vi "FilesIOex1.vi"() -> ()   [LabVIEW 2015]
panel:
  in  "access (0:read/write)":enum16{"read/write", "read-only", "write-only"}(ring)
  in  "operation (0:open)":T1(ring)
  in  "stop":bool
  in  "file path (use dialog)":path
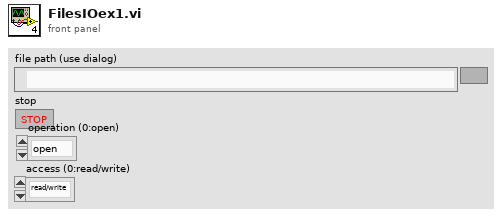
[diagram p1: front panel]
types:
  T1 = enum16{"open", "replace", "create", "open or create", "replace or create", "replace or create with confirmation"}
  T2 = enum16{"Native", "Native Command Line", "UNIX", "Macintosh", "DOS"}
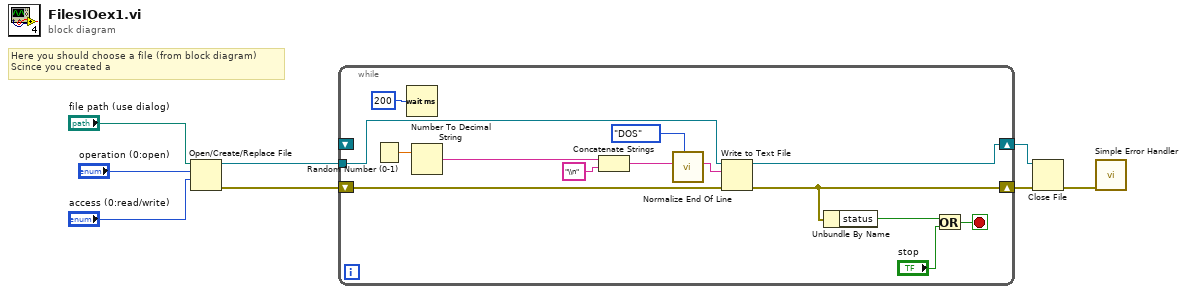
[diagram p0: block diagram]
diagram:
  # "Here you should choose a file (from block diagram)\nScince you created a"
  n1 = Open/Create/Replace File(file path (use dialog)="file path (use dialog)", operation (0:open)="operation (0:open)", access (0:read/write)="access (0:read/write)") -> (refnum out=w7:refnum<file>, error out=w6:errorcluster)  [unwired: 3 in, 1 out]
  n2 = while {
    tunnel: w7 -> [w18]
    shift-right: [w17] -> w4
    shift-left: _ -> [_]
    shift-right: [w15] -> w5
    shift-left: w6 -> [w16]
    stop <- w22 stop-if-true
    n3 = Random Number (0-1)() -> (number: 0 to 1=w19:dbl)
    n4 = Wait (ms)(milliseconds to wait=u32 200) -> ()  [unwired: 1 out]
    n5 = Number To Decimal String(number=w19) -> (decimal integer string=w10:string)  [unwired: 1 in]
    n6 = Concatenate Strings(w10, "\\n") -> (w11:string)
    n7 = call <vilib>:"Normalize End Of Line.vi"("end of line (Native)"=T2."DOS", "string in"=w11) -> ("string out"=w13:string)  [unwired: 6 in]
    n8 = Write to Text File(file (use dialog)=w18, text=w13, error in=w16) -> (refnum out=w17:refnum<file>, error out=w15:errorcluster)  [unwired: 1 in, 1 out]
    n9 = Unbundle By Name "Unbundle By Name"(w15) -> ("status"=w21:bool)
    n10 = Or(x=w21, y="stop") -> (x .or. y?=w22:bool)
  }
  n11 = Close File(refnum=w4, error in=w5) -> (error out=w3:errorcluster)  [unwired: 1 out]
  n12 = call <vilib>:"Simple Error Handler.vi"("error in (no error)"=w3) -> ()  [unwired: 4 in, 5 out]
